vi "MQTT_Unsubscribe.vi"(8 "error in (no error)":errorcluster, 9 "Message ID":u16=10 format="%x", 10 "UnSubscribe Topic Array":string[](array[string]), 11 "connection ID":refnum<k5>) -> (0 "error out":errorcluster, 2 "Unsubscribe Message":u8[](array[numeric]) format="%x", 3 "connection ID out":refnum<k5>)   [LabVIEW 2013, in "MQTT_Functions.lvlib"]
doc: "This VI unsubscribes the client from a topic. The client can no longer read published messages for the topic. \n\n© 2015 - daq.io, LLC - Peter Adelhardt"
uses:
  MQTT_Functions.lvlib
  Controls/MessageType.ctl
  Controls/Retain_Flag.ctl
  Controls/DUP_Flag.ctl
  Controls/QoS.ctl
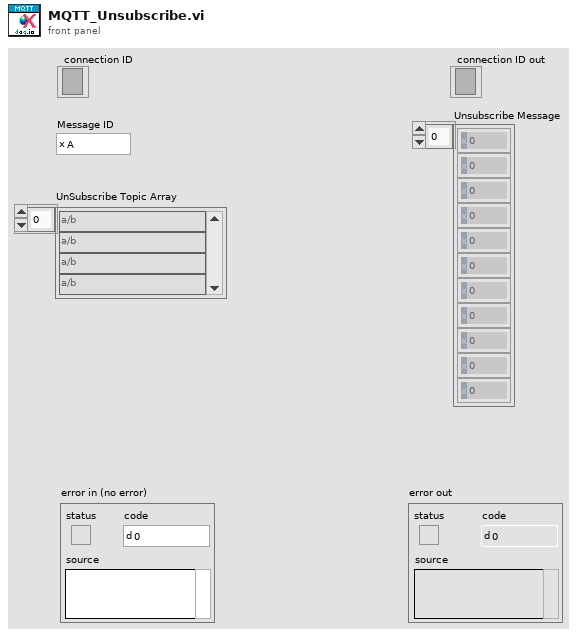
[diagram p1: front panel]
types:
  T1 = typedef "MQTT_Functions.lvlib/QoS.ctl" = enum8{"At most once", "At least once", "Exactly once", "Reserved"}
  T2 = typedef "MQTT_Functions.lvlib/DUP_Flag.ctl" = bool
  T3 = typedef "MQTT_Functions.lvlib/Retain_Flag.ctl" = bool
  T4 = typedef "MQTT_Functions.lvlib/MessageType.ctl" = enum32{"Reserved", "CONNECT", "CONNACK", "PUBLISH", "PUBACK", "PUBREC", "PUBREL", "PUBCOMP", "SUBSCRIBE", "SUBACK", "UNSUBSCRIBE", "UNSUBACK", "PINGREQ", "PINGRESP", "DISCONNECT", "Reserved2"}
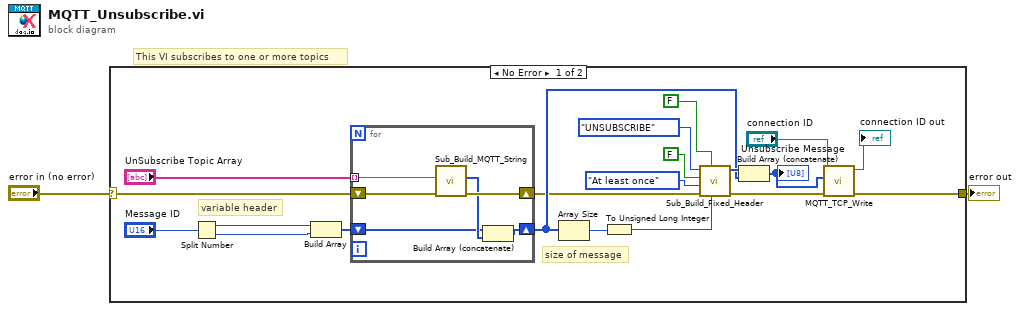
[diagram p0: block diagram]
diagram:
  # "This VI subscribes to one or more topics"
  n1 = case shown="No Error" "error in (no error)" {
    selector: "error in (no error)" -> [w15 w29]
    tunnel: [w6 w29] -> w1
    frame No Error {
      # "variable header"
      # "size of message"
      n2 = Split Number(x="Message ID") -> (hi(x)=w18:u8, lo(x)=w17:u8)
      n3 = Build Array(w18, w17) -> (w12:u8[])
      n4 = for {
        tunnel: "UnSubscribe Topic Array" -> [w23] mode=indexing
        shift-right: [w27] -> w8
        shift-left: w15 -> [w28]
        shift-right: [w25] -> w14
        shift-left: w12 -> [w24]
        n5 = call "Sub_Build_MQTT_String.vi"("error in (no error)"=w28, "String to be encoded"=w23) -> ("error out"=w27:errorcluster, "UTF8 Byte Array"=w26:u8[])  [unwired: 8 in]
        n6 = Build Array (concatenate)(w24, w26) -> (w25:u8[])
      }
      n7 = Array Size(array=w14) -> (size(s)=w20:i32)
      n8 = To Unsigned Long Integer(number=w20) -> (unsigned 32bit integer=w21:u32)
      n9 = call "Sub_Build_Fixed_Header.vi"("Remaining Length"=w21, "Retain"=T3 FALSE, "error in (no error)"=w8, "QoS"=QoS."At least once", "DUP"=T2 FALSE, "MessageType"=MessageType."UNSUBSCRIBE") -> ("error out"=w7:errorcluster, "Fixed Header"=w19:u8[])  [unwired: 4 in]
      n10 = Build Array (concatenate)(w19, w14) -> (w3:u8[])
      "Unsubscribe Message" <- w3
      n11 = call "MQTT_TCP_Write.vi"("error in (no error)"=w7, "data in"=w3, "connection ID"="connection ID") -> ("error out"=w6:errorcluster, "connection ID out"=→"connection ID out":refnum<k5>)  [unwired: 6 in, 1 out]
    }
    frame Error {
    }
  }
  "error out" <- w1
